vi "driveController.vi"(1 "Max. Speed":dbl=0.12, 2 "Stop?":bool, 3 "currentSpeed":cluster{"left":dbl, "right":dbl}={"left"=1.0000000000000004, "right"=1.0000001911095793}, 4 "inputSpeed":cluster{"left":dbl, "right":dbl}) -> (0 "outputSpeed":cluster{"left":dbl, "right":dbl}={"left"=0.7500000000000003, "right"=0.7500001433321845})   [LabVIEW 2016]
uses:
  <vilib>/myRIO/Instrument Drivers/Onboard IO/PWM/typedefs/PWM Reference.ctl
  <vilib>/myRIO/Common/Instrument Driver Framework/Utilities/typedefs/myRIO Generic Hardware Reference.ctl
  <vilib>/myRIO/Common/Instrument Driver Framework/Utilities/typedefs/Hardware Version Enum.ctl
  <vilib>/myRIO/Common/Instrument Driver Framework/Utilities/typedefs/myRIO v1.0 Reference.ctl
  <vilib>/myRIO/Common/Instrument Driver Framework/Utilities/typedefs/Generic FPGA Reference.ctl
  <vilib>/myRIO/Common/Instrument Driver Framework/myRIO v1.0/PWM/typedefs/PWM Channels Enum.ctl
  <vilib>/myRIO/Instrument Drivers/Onboard IO/PWM/typedefs/PWM Configuration.ctl
  <vilib>/userdefined/High Color/nirio_resource_hc.ctl
  <vilib>/myRIO/Common/Instrument Driver Framework/Utilities/vis/Is FPGA Ref Available.vi
  <vilib>/myRIO/Common/Instrument Driver Framework/myRIO v1.0/PWM/vis/myRIO v1.1 Open PWM.vi
  <vilib>/myRIO/Instrument Drivers/Onboard IO/PWM/vis/Set Duty Cycle and Frequency.vi
  <vilib>/myRIO/Common/Instrument Driver Framework/Utilities/vis/Validate Channels.vi
  <vilib>/myRIO/Common/Instrument Driver Framework/myRIO v1.0/PWM/vis/myRIO v1.0 Reserve PWM.vi
  <vilib>/myRIO/Common/Instrument Driver Framework/myRIO v1.0/PWM/vis/myRIO v1.0 Build MUX Configuration PWM.vi
  <vilib>/myRIO/Common/Instrument Driver Framework/myRIO v1.0/Resource Manager/vis/myRIO v1.0 Reserve Channel List.vi
  <vilib>/myRIO/Common/Instrument Driver Framework/myRIO v1.0/Resource Manager/vis/myRIO v1.0 Create Configuration List.vi
  <vilib>/myRIO/Common/Instrument Driver Framework/myRIO v1.0/Resource Manager/vis/myRIO v1.0 Reserve Channel.vi
  <vilib>/myRIO/Common/Instrument Driver Framework/myRIO v1.0/Resource Manager/vis/myRIO v1.0 Unreserve Channel.vi
  <vilib>/myRIO/Common/Instrument Driver Framework/myRIO v1.0/Resource Manager/vis/myRIO v1.0 Build Mutex Name.vi
  <vilib>/Utility/VariantDataType/GetNumericInfo.vi
  <vilib>/Utility/error.llb/Error Cluster From Error Code.vi
  <vilib>/myRIO/Common/Instrument Driver Framework/myRIO v1.0/myRIO v1.1 Open.vi
  <vilib>/myRIO/Common/Instrument Driver Framework/Utilities/vis/IO Manager.vi
  <vilib>/myRIO/Common/Instrument Driver Framework/Utilities/vis/Configuration Manager.vi
  <vilib>/myRIO/Common/Instrument Driver Framework/myRIO v1.0/Resource Manager/vis/myRIO v1.0 Configure IO.vi
  <vilib>/myRIO/Common/Instrument Driver Framework/myRIO v1.0/myRIO v1.0 Close.vi
  <vilib>/myRIO/Common/Instrument Driver Framework/myRIO v1.0/PWM/vis/myRIO v1.0 Write PWM.vi
  <vilib>/myRIO/Express VI/Onboard IO/PWM/PWM Express VI.xnode
  <vilib>/myRIO/Instrument Drivers/Onboard IO/PWM/vis/myRIO PWM Open.xnode
  <vilib>/myRIO/Instrument Drivers/Onboard IO/PWM/PWM.lvlib
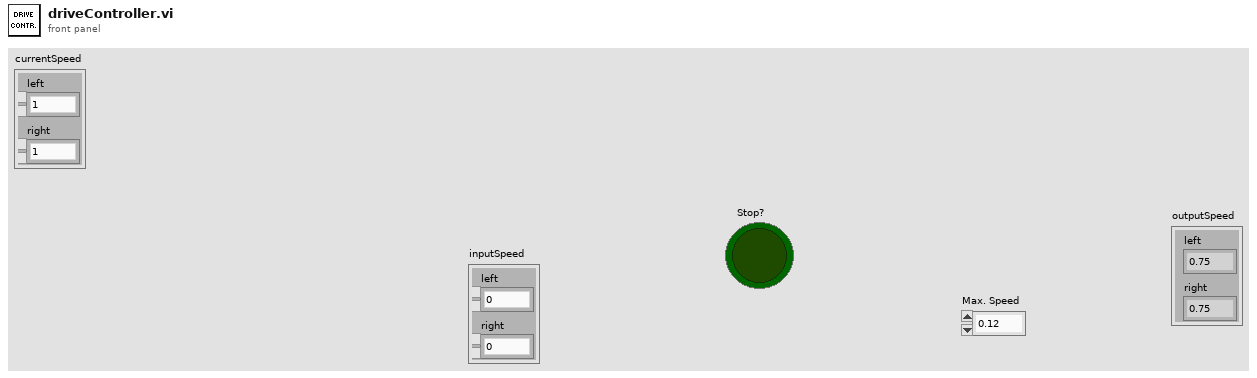
[diagram p1: front panel]
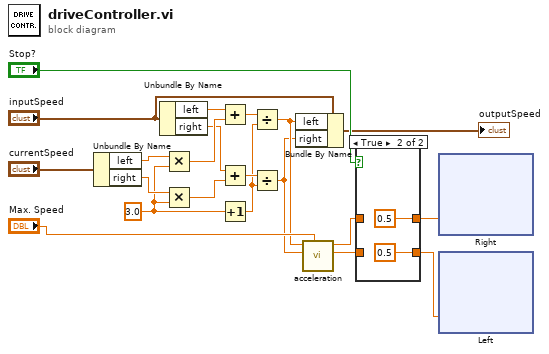
[diagram p0: block diagram]
diagram:
  w1 = 3.0 ("y")
  n1 = Unbundle By Name("currentSpeed") -> ("left"=w10:dbl, "right"=w5:dbl)
  n2 = Unbundle By Name("inputSpeed") -> ("left"=w12:dbl, "right"=w6:dbl)
  n3 = Multiply(x=w10, y=w1) -> (x*y=w9:dbl)
  n4 = Multiply(x=w5, y=w1) -> (x*y=w7:dbl)
  n5 = Add(x=w12, y=w9) -> (x+y=w13:dbl)
  n6 = Add(x=w6, y=w7) -> (x+y=w8:dbl)
  n7 = Increment(x=w1) -> (x+1=w2:dbl)
  n8 = Divide(x=w13, y=w2) -> (x/y=w4:dbl)
  n9 = Divide(x=w8, y=w2) -> (x/y=w3:dbl)
  n10 = Bundle By Name(cluster="inputSpeed", "left"=w4, "right"=w3) -> (→"outputSpeed":cluster{"left":dbl, "right":dbl})
  n11 = call "acceleration.vi"("Max. Speed"="Max. Speed", "Right"=w3, "Left"=w4) -> ("PWM right"=w18:dbl, "PWM left"=w19:dbl)  [unwired: 7 in]
  n12 = case shown="True" "Stop?" {
    tunnel: [w22 0.5] -> w21
    tunnel: [w23 0.5] -> w20
    tunnel: w19 -> [w23 _]
    tunnel: w18 -> [w22 _]
    frame False {
    }
    frame True {
    }
  }
  n13 = xnode "Right"("Duty Cycle"=w20) -> ()  [unwired: 1 in, 1 out]
  n14 = xnode "Left"("Duty Cycle"=w21) -> ()  [unwired: 1 in, 1 out]
